vi "HXG2_Programmer-Save.vi"(6 "Inteval Show?":bool, 8 "error In":errorcluster, 10 "Quit? In":bool, 11 "Save? In":bool) -> (0 "error Out":errorcluster, 2 "Quit? Out":bool, 3 "Save? Out":bool, 4 "Inteval Show?":bool)   [LabVIEW 2012]
doc: "Saves if programmer is running and save data is true\n\nAND if Programmer state is running and interval is true"
uses:
  Modules/Programmer/HXG2programmer.ctl
  Modules/Programmer/Data Types/Programmer Execution States.ctl
  Modules/Programmer/Data Types/Programmer State.ctl
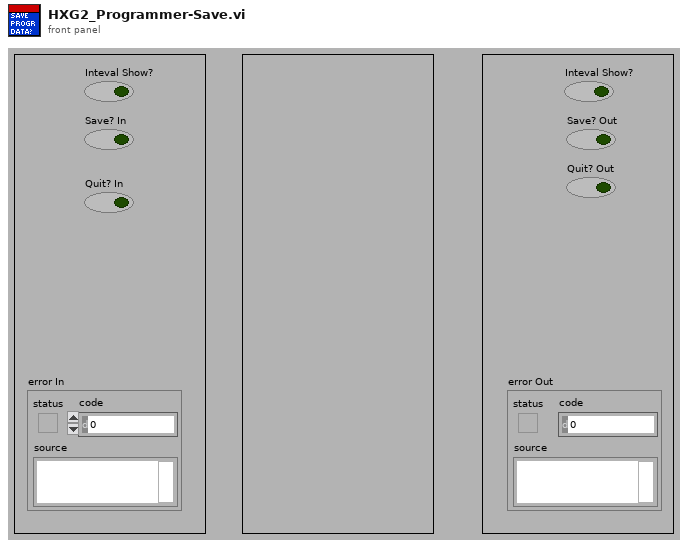
[diagram p1: front panel]
types:
  T1 = typedef "HXG2programmer.ctl" = enum16{"Write Refs", "Write Selec", "Write All", "Pass All", "React", "Write Path"}
  T2 = typedef "HXG2programmerUserSelections.ctl" = cluster{"Run Prog":bool, "Done Stop":bool, "Load Profile":bool, "Save Profile":bool, "Repeat Execution:":i32, "Start Programmer":bool, "Stop Programmer":bool}
  T3 = typedef "Programmer State.ctl" = enum16{"Prepare Next Test Step", "Stopped", "Running", "Stabilizing"}
  T4 = typedef "Programmer Execution States.ctl" = enum16{"Register Steps", "Initialize", "Start Test Sequence", "Register Data", "Execute Programmer", "Set Number of Repetitions", "Get Current Step Index", "Get Time Until Step Ends"}
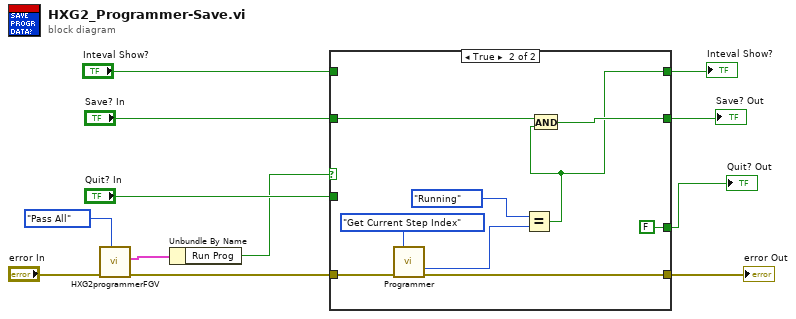
[diagram p0: block diagram]
diagram:
  n1 = call "HXG2programmerFGV.vi"("Programmer Ctrl"=HXG2programmer."Pass All", "error in (no error)"="error In") -> ("error out"=w6:errorcluster, "User Selections Out"=w4:T2)  [unwired: 5 in, 3 out]
  n2 = Unbundle By Name(w4) -> ("Run Prog"=w3:bool)
  n3 = case shown="True" w3 {
    tunnel: [w16 w18] -> w9
    tunnel: "Save? In" -> [w16 w19]
    tunnel: [w15 FALSE ("Quit? In")] -> w10
    tunnel: "Quit? In" -> [w15 _]
    tunnel: [w14 w23] -> w8
    tunnel: w6 -> [w14 w24]
    tunnel: "Inteval Show?" -> [w13 _]
    tunnel: [w13 w17] -> w1
    frame False {
    }
    frame True {
      n4 = call "Programmer.vi"("Action"=Programmer_Execution_States."Get Current Step Index", "error in (no error)"=w24) -> ("Programmer State"=w21:T3, "error out"=w23:errorcluster)  [unwired: 6 in, 6 out]
      n5 = Equal?(x=Programmer_State."Running" ("Programmer State"), y=w21) -> (x = y?=w17:bool)
      n6 = And(x=w19, y=w17) -> (x .and. y?=w18:bool)
    }
  }
  "Save? Out" <- w9
  "Quit? Out" <- w10
  "error Out" <- w8
  "Inteval Show?" <- w1
